vi "Centre Window.vi"(7 "Parent Window":refnum<class "Window.lvclass">, 8 "error in (no error)":errorcluster, 11 "Window in":refnum<class "Window.lvclass">) -> (0 "error out":errorcluster, 3 "Window out":refnum<class "Window.lvclass">)   [LabVIEW 2015, in "IBEX Device.lvlib" / "Window.lvclass"]
doc: "Move the child window to the centre of the same monitor as the parent window."
uses:
  Window.lvclass
  Window.lvclass/Window.ctl
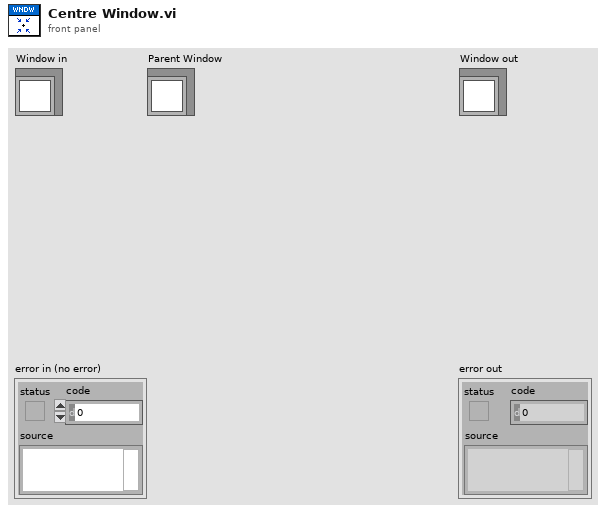
[diagram p1: front panel]
types:
  T1 = enum32{"Invalid", "Standard", "Closed", "Hidden", "Minimized", "Maximized"}
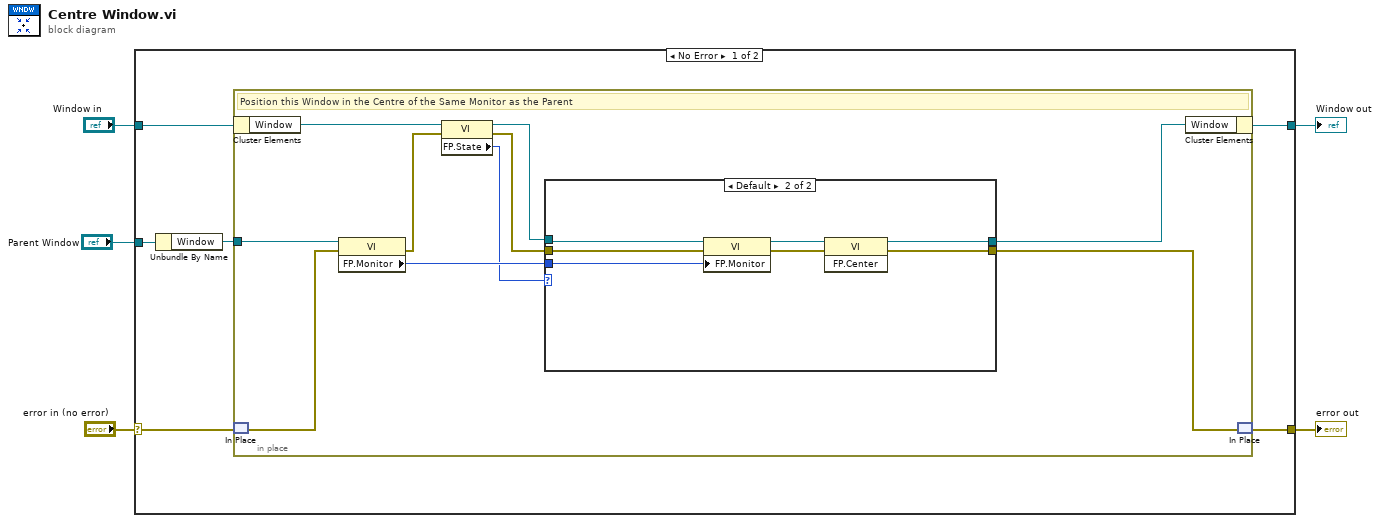
[diagram p0: block diagram]
diagram:
  n1 = case shown="No Error" "error in (no error)" {
    selector: "error in (no error)" -> [w9 w32]
    tunnel: [w8 w32] -> w4
    tunnel: [w10 w31] -> w2
    tunnel: "Window in" -> [w6 w31]
    tunnel: "Parent Window" -> [w7 _]
    frame No Error {
      n2 = Unbundle By Name(w7) -> ("Window"=w11:refnum<vi>)
      n3 = in-place {
        in-place-border: w11 -> [w18]
        # "Position this Window in the Centre of the Same Monitor as the Parent"
        n4 = in-place-cluster #1(w6) -> ("Window"=w17:refnum<vi>)
        n5 = in-place-match #2(w9) -> (w21:errorcluster)
        n6 = property class="VI"(reference=w18, error in=w21) -> (error out=w14:errorcluster, "FP.Monitor"=w20:u16)  [unwired: 1 out]
        n7 = property class="VI"(reference=w17, error in=w14) -> (reference out=w15:refnum<vi>, error out=w13:errorcluster, "FP.State"=w12:T1)
        n8 = case shown="Default" w12 {
          tunnel: w13 -> [w23 w30]
          tunnel: w20 -> [_ w29]
          tunnel: [w23 w28] -> w19
          tunnel: w15 -> [w22 w27]
          tunnel: [w22 w26] -> w16
          frame "Invalid", "Closed" {
          }
          frame Default {
            n9 = property class="VI"(reference=w27, error in=w30, "FP.Monitor"=w29) -> (reference out=w24:refnum<vi>, error out=w25:errorcluster)
            n10 = invoke class="VI" method="FP.Center"(reference=w24, error in=w25) -> (reference out=w26:refnum<vi>, error out=w28:errorcluster)  [unwired: 1 in, 1 out]
          }
        }
        n11 = in-place-cluster #1("Window"=w16) -> (w10:refnum<class "Window.lvclass">)
        n12 = in-place-match #2(w19) -> (w8:errorcluster)
      }
    }
    frame Error {
    }
  }
  "error out" <- w4
  "Window out" <- w2
